vi "Add Property.vi"(6 "Property Name":string, 9 "Setter":refnum<vi>, 10 "Getter":refnum<vi>, 11 "Class":refnum<vi>) -> (3 "Class Dup":refnum<vi>)   [LabVIEW 2013]
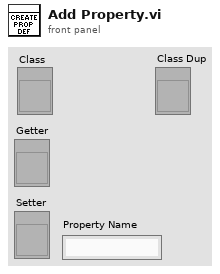
[diagram p1: front panel]
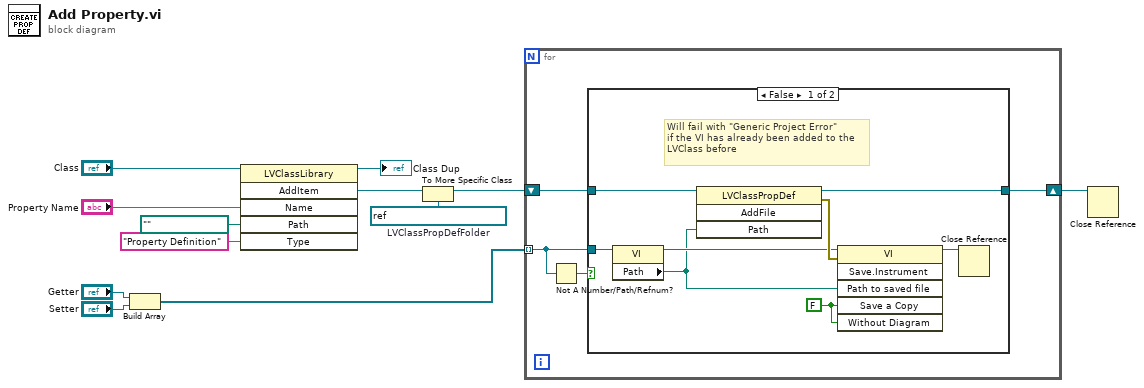
[diagram p0: block diagram]
diagram:
  w8 = refnum<vi> refnum  # LVClassPropDefFolder
  n1 = Build Array("Getter", "Setter") -> (w3:refnum<vi>[])
  n2 = invoke class="LVClassLibrary" method="AddItem"(reference="Class", "Name"="Property Name", "Path"=path "", "Type"="Property Definition") -> (reference out=→"Class Dup":refnum<vi>, "AddItem"=w9:refnum<vi>)  [unwired: 2 in, 4 out]
  n3 = To More Specific Class(target class=w8, reference=w9) -> (specific class reference=w2:refnum<vi>)  [unwired: 1 in, 1 out]
  n4 = for {
    tunnel: w3 -> [w15] mode=indexing
    shift-right: [w13] -> w1
    shift-left: w2 -> [w14]
    n5 = Not A Number/Path/Refnum?(number/path/refnum=w15) -> (NaN/Path/Refnum?=w16:bool)
    n6 = case shown="False" w16 {
      tunnel: w15 -> [w24 _]
      tunnel: w14 -> [w23 w25]
      tunnel: [w17 w25] -> w13
      frame False {
        w19 = FALSE ("Save a Copy")
        # "Will fail with \"Generic Project Error\"\nif the VI has already been added to the\nLVClass before"
        n7 = property class="VI"(reference=w24) -> (reference out=w21:refnum<vi>, "Path"=w20:path)  [unwired: 1 in, 1 out]
        n8 = invoke class="LVClassPropDef" method="AddFile"(reference=w23, "Path"=w20) -> (reference out=w17:refnum<vi>, error out=w22:errorcluster)  [unwired: 2 in, 2 out]
        n9 = invoke class="VI" method="Save.Instrument"(reference=w21, error in=w22, "Path to saved file"=w20, "Save a Copy"=w19, "Without Diagram"=w19) -> (reference out=w18:refnum<vi>)  [unwired: 1 in, 5 out]
        n10 = Close Reference(reference=w18) -> ()  [unwired: 1 in, 1 out]
      }
      frame True {
      }
    }
  }
  n11 = Close Reference(reference=w1) -> ()  [unwired: 1 in, 1 out]
